vi "Get Library from This Project.vi"(8 "error in (no error)":errorcluster, 10 "Target Name (My Computer)":string="My Computer", 11 "Library Name":string) -> (0 "error out":errorcluster, 3 "Library Refnum":refnum<vi>)   [LabVIEW 2020, in "Build Automation.lvlib"]
uses:
  Build Automation.lvlib
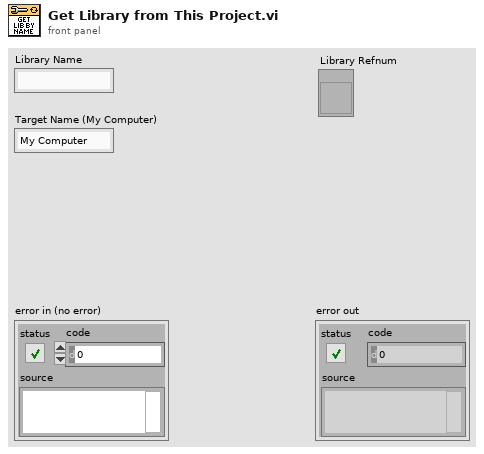
[diagram p1: front panel]
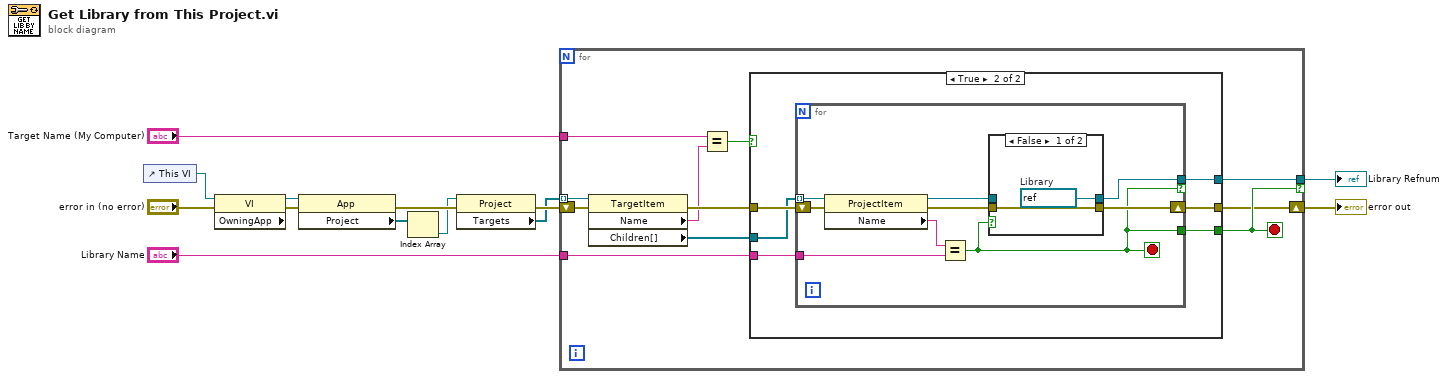
[diagram p0: block diagram]
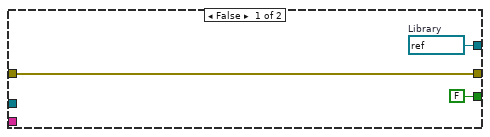
[diagram p2: hidden frame]
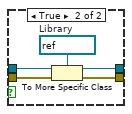
[diagram p3: hidden frame]
diagram:
  n1 = control-ref of="This VI"() -> (w13:refnum<vi>)
  n2 = property class="VI"(reference=w13, error in="error in (no error)") -> (error out=w4:errorcluster, "OwningApp"=w12:refnum<vi>)  [unwired: 1 out]
  n3 = property class="App"(reference=w12, error in=w4) -> (error out=w6:errorcluster, "Project"=w11:refnum<vi>[])  [unwired: 1 out]
  n4 = Index Array(array=w11) -> (element=w5:refnum<vi>)  [unwired: 1 in]
  n5 = property class="Project"(reference=w5, error in=w6) -> (error out=w3:errorcluster, "Targets"=w2:refnum<vi>[])  [unwired: 1 out]
  n6 = for {
    tunnel: w2 -> [w24] mode=indexing
    tunnel: "Library Name" -> [w23]
    tunnel: [w22] -> w9 if=w21
    shift-right: [w20] -> w7
    shift-left: w3 -> [w19]
    tunnel: "Target Name (My Computer)" -> [w15]
    stop <- w21 stop-if-true
    n7 = property class="TargetItem"(reference=w24, error in=w19) -> (error out=w18:errorcluster, "Name"=w16:string, "Children[]"=w17:refnum<vi>[])  [unwired: 1 out]
    n8 = Equal?(x=w15, y=w16) -> (x = y?=w14:bool)
    n9 = case shown="True" w14 {
      tunnel: w23 -> [_ w33]
      tunnel: [w27 w32] -> w22
      tunnel: [FALSE w31] -> w21
      tunnel: [w25 w30] -> w20
      tunnel: w18 -> [w25 w29]
      tunnel: w17 -> [_ w28]
      frame False {
        w27 = refnum<vi> refnum  # Library
      }
      frame True {
        n10 = for {
          tunnel: w28 -> [w42] mode=indexing
          tunnel: w33 -> [w40]
          tunnel: [w36] -> w32 if=w34
          shift-right: [w38] -> w30
          shift-left: w29 -> [w35]
          tunnel: [w34] -> w31
          stop <- w34 stop-if-true
          n11 = property class="ProjectItem"(reference=w42, error in=w35) -> (reference out=w37:refnum<vi>, error out=w39:errorcluster, "Name"=w41:string)
          n12 = Equal?(x=w41, y=w40) -> (x = y?=w34:bool)
          n13 = case shown="False" w34 {
            tunnel: w39 -> [w44 w49]
            tunnel: [w44 w48] -> w38
            tunnel: w37 -> [_ w47]
            tunnel: [w43 w46] -> w36
            frame False {
              w43 = refnum<vi> refnum  # Library
            }
            frame True {
              w45 = refnum<vi> refnum  # Library
              n14 = To More Specific Class(target class=w45, reference=w47, error in=w49) -> (specific class reference=w46:refnum<vi>, error out=w48:errorcluster)
            }
          }
        }
      }
    }
  }
  "Library Refnum" <- w9
  "error out" <- w7
